vi "UNIX Timer To LabView Timer.vi"() -> ()   [LabVIEW 2018]
panel:
  out "LabVIEW时间标识":timestamp
  in  "UNIX时间戳":u64
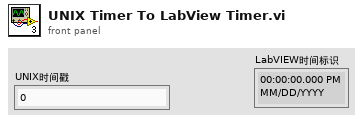
[diagram p1: front panel]
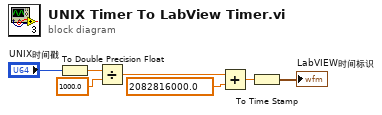
[diagram p0: block diagram]
diagram:
  n1 = To Double Precision Float(number="UNIX时间戳") -> (double precision float=w7:dbl)
  n2 = Divide(x=w7, y=1000.0) -> (x/y=w5:dbl)
  n3 = Add(x=w5, y=2082816000.0 ("双精度浮点数")) -> (x+y=w3:dbl)
  n4 = To Time Stamp(1:w3) -> (0:→"LabVIEW时间标识":timestamp)
